vi "WaitUntilStatus.vi"(8 "check interval (ms)":dbl, 11 "target status":string) -> ()   [LabVIEW 2018]
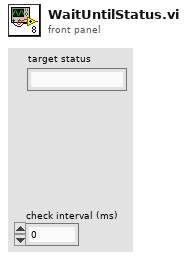
[diagram p1: front panel]
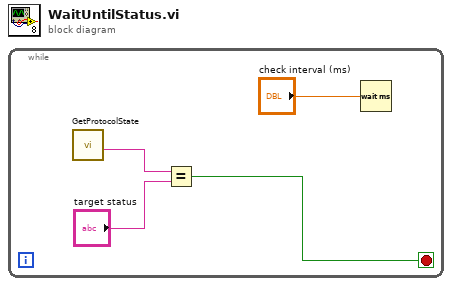
[diagram p0: block diagram]
diagram:
  n1 = while {
    stop <- w2 stop-if-true
    n2 = call "GetProtocolState.vi"() -> ("state"=w3:string)  [unwired: 11 in]
    n3 = Equal?(x=w3, y="target status") -> (x = y?=w2:bool)
    n4 = Wait (ms)(milliseconds to wait="check interval (ms)") -> ()  [unwired: 1 out]
  }
